vi "RMStoreFrameInfo.vi"(0 "ResultManager":T1, 5 "timestamp":dbl, 7 "frame":i32, 9 "columns":sgl[](array[numeric]), 11 "error in (no error)":errorcluster) -> (4 "ResultManager (out)":T1, 15 "error out":errorcluster)   [LabVIEW 2011]
uses:
  ResultManagerInstance.ctl
  QTrkDLL.vi
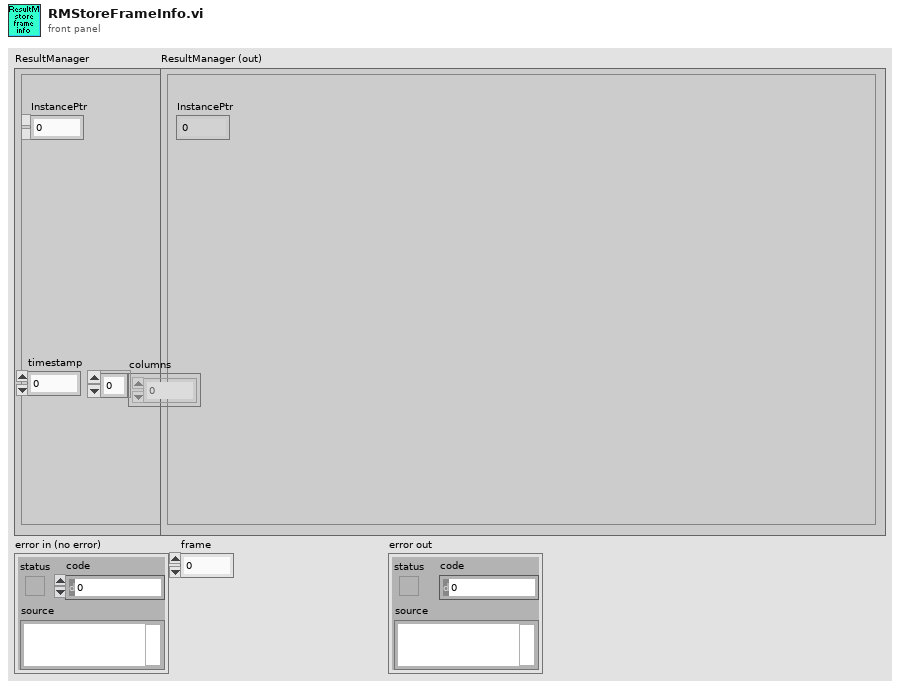
[diagram p1: front panel]
types:
  T1 = typedef "ResultManagerInstance.ctl" = cluster{"InstancePtr":u64}
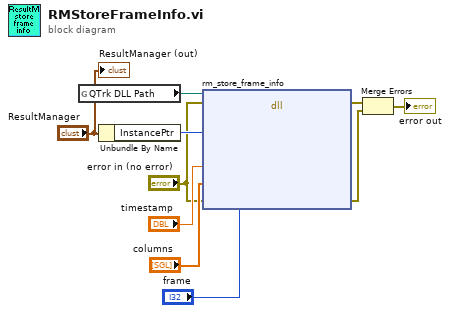
[diagram p0: block diagram]
diagram:
  n1 = global read "QTrkDLL.vi" "QTrk DLL Path"() -> (w6:path)
  n2 = Unbundle By Name("ResultManager") -> ("InstancePtr"=w9:u64)
  n3 = dll-call lib="D:/jcnossen1/cudaqi-tracker/bin/jtrk-labview.dll" fn="rm_store_frame_info"(path in=w6, error in="error in (no error)", "resultmanager"=w9, "frame"="frame", "timestamp"="timestamp", "columns"="columns", "error"="error in (no error)") -> (error out=w4:errorcluster, "error"=w3:errorcluster)  [unwired: 6 in, 1 out]
  n4 = Merge Errors(w4, w3) -> (→"error out":errorcluster)
  "ResultManager (out)" <- "ResultManager"
